vi "Finalize.vi"(8 "error in":errorcluster, 11 "Plugin in":refnum<class "Test Sequencer.lvclass">) -> (0 "error out":errorcluster, 3 "Plugin out":refnum<class "Test Sequencer.lvclass">)   [LabVIEW 2020, in "Test Sequencer.lvlib" / "Test Sequencer.lvclass"]
uses:
  Test Sequencer.lvclass
  Test Sequencer.lvclass/Test Sequencer.ctl
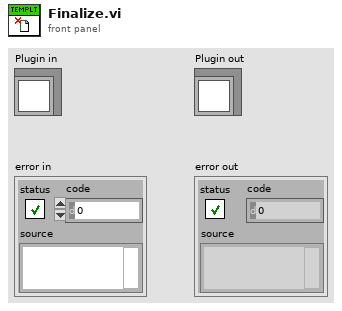
[diagram p1: front panel]
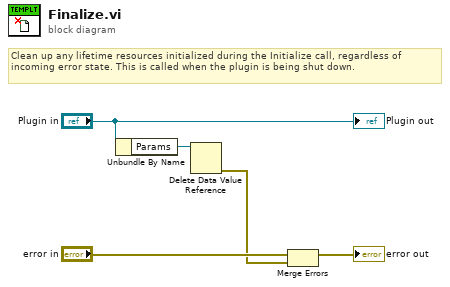
[diagram p0: block diagram]
diagram:
  # "Clean up any lifetime resources initialized during the Initialize call, regardless of incoming error state. This is called when the plugin is being shut down."
  n1 = Unbundle By Name("Plugin in") -> ("Params"=w2:refnum<data-value>)
  n2 = Delete Data Value Reference(data value reference=w2) -> (error out=w1:errorcluster)  [unwired: 1 in, 1 out]
  n3 = Merge Errors("error in", w1) -> (→"error out":errorcluster)
  "Plugin out" <- "Plugin in"
